vi "ELVIS III v1.0 AO Block Write Resource Manager.vi"(5 "DMA Resource":u8, 7 "Action":enum16{"Set", "Get"}(ring), 8 "error in (no error)":errorcluster, 10 "AO Resource In":T1={"AO FIFO Clock Divisor"=1000, "Wait Until Done?"=TRUE, "Write Mode"=0, "AO (N Samples) Configuration "=[]} caption="DO (N Samples) Configuration") -> (0 "error out":errorcluster, 1 "Action Succeeds":bool, 2 "AO Resource Out":T1={"AO FIFO Clock Divisor"=1000, "Wait Until Done?"=TRUE, "Write Mode"=0, "AO (N Samples) Configuration "=[]} caption="DO (N Samples) Configuration")   [LabVIEW 2021]
uses:
  <vilib>/myRIO/Common/Instrument Driver Framework/ELVIS III v1.0/AO Block/typedefs/ELVIS III AO Block Configuration.ctl
  <vilib>/myRIO/Common/Instrument Driver Framework/ELVIS III v1.0/AO Block/typedefs/ELVIS III AO Block Bank Data.ctl
  <vilib>/myRIO/Common/Instrument Driver Framework/myRIO v1.0/Resource Manager/vis/myRIO v1.0 Block Write Configuration.vi
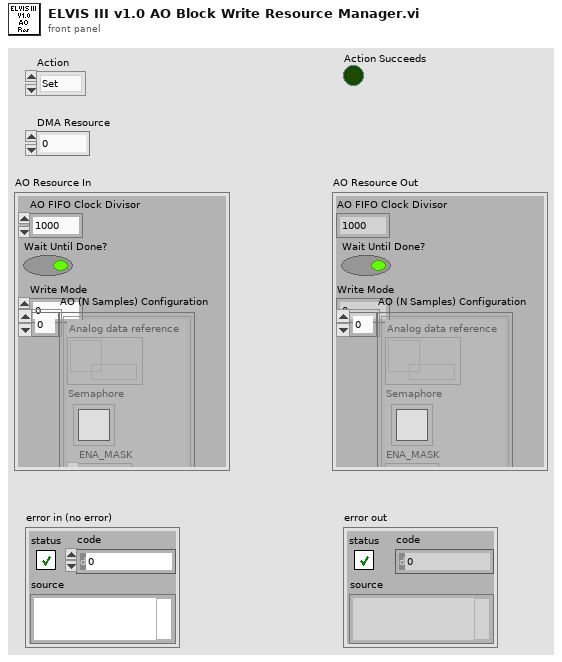
[diagram p1: front panel]
types:
  T1 = typedef "ELVIS III AO Block Configuration.ctl" = cluster{"AO FIFO Clock Divisor":u32, "Wait Until Done?":bool, "Write Mode":u8, "AO (N Samples) Configuration ":T2[]}
  T2 = typedef "ELVIS III AO Block Bank Data.ctl" = cluster{"Analog data reference":refnum<data-value>, "Semaphore":T3, "ENA_MASK":u8}
  T3 = typedef "Semaphore RefNum" = refnum<k1>
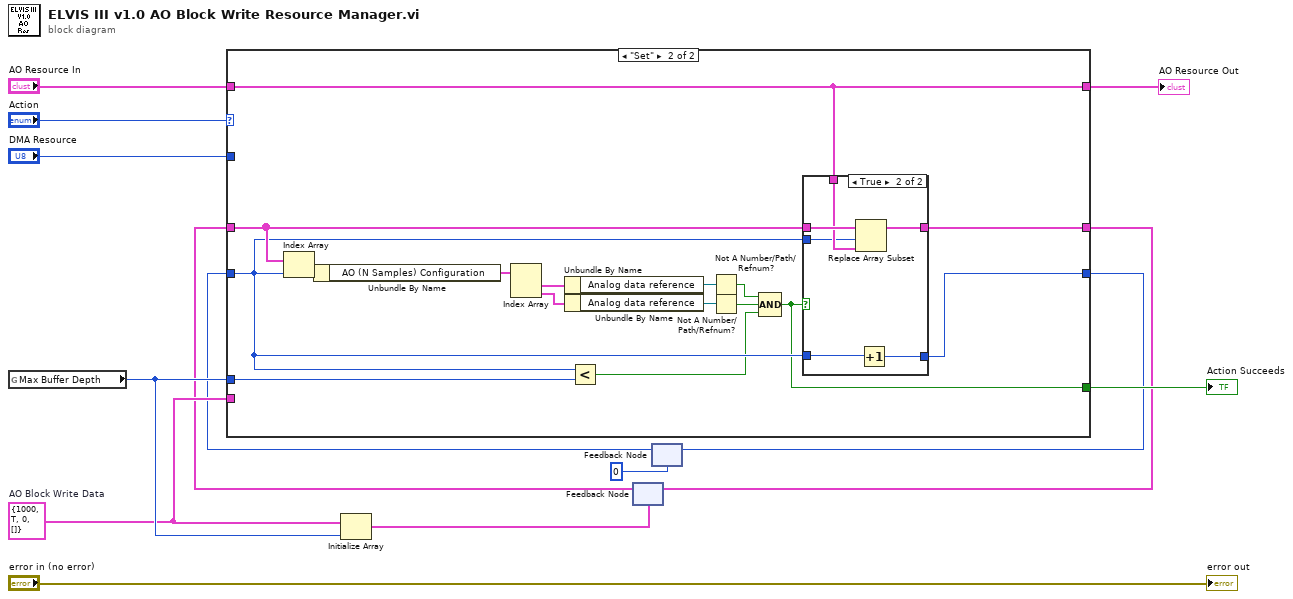
[diagram p0: block diagram]
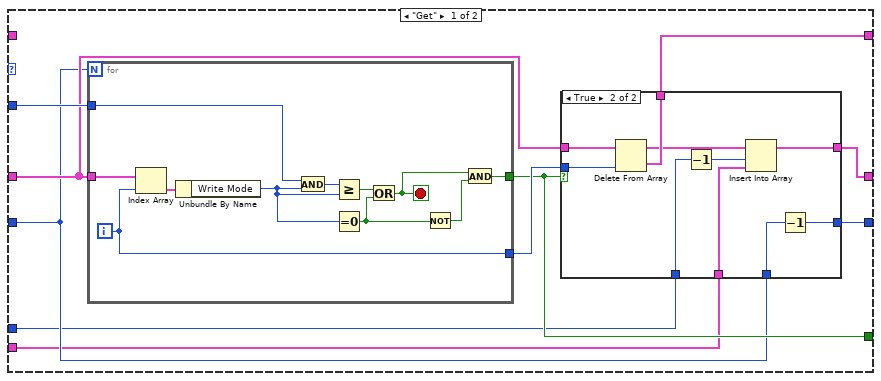
[diagram p2: hidden frame]
diagram:
  w10 = T1 {"AO FIFO Clock Divisor"=1000, "Wait Until Done?"=TRUE, "Write Mode"=0, "AO (N Samples) Configuration "=[]}  # AO Block Write Data
  n1 = global read "myRIO v1.0 Block Write Configuration.vi" "Max Buffer Depth"() -> (w13:u32)
  n2 = Initialize Array(w10, w13) -> (w6:T1[])
  n3 = feedback #1(w6) -> (w7:T1[])
  n4 = feedback #2(0) -> (w3:i32)
  n5 = case shown="\"Set\"" "Action" {
    tunnel: [w21 w57] -> w5
    tunnel: w7 -> [w22 w56]
    tunnel: "AO Resource In" -> [_ w52]
    tunnel: [w17 w55] -> w4
    tunnel: w13 -> [w16 w50]
    tunnel: w3 -> [w18 w51]
    tunnel: [w20 w48] -> w11
    tunnel: [w19 w52] -> w1
    tunnel: w10 -> [w15 _]
    tunnel: "DMA Resource" -> [w24 _]
    frame "Get" {
      n6 = for {
        N: w18 -> [_]
        tunnel: w22 -> [w46]
        tunnel: w24 -> [w45]
        tunnel: [w43] -> w23
        tunnel: [w38] -> w20
        i -> [w43]
        stop <- w40 stop-if-true
        n7 = Index Array(array=w46, index=w43) -> (element=w47:T1)
        n8 = Unbundle By Name(w47) -> ("Write Mode"=w42:u8)
        n9 = And(x=w45, y=w42) -> (x .and. y?=w37:u8)
        n10 = Greater Or Equal?(x=w37, y=w42) -> (x >= y?=w44:bool)
        n11 = Equal To 0?(x=w42) -> (x = 0?=w41:bool)
        n12 = Or(x=w44, y=w41) -> (x .or. y?=w40:bool)
        n13 = Not(x=w41) -> (.not. x?=w39:bool)
        n14 = And(x=w40, y=w39) -> (x .and. y?=w38:bool)
      }
      n15 = case shown="True" w20 {
        tunnel: w23 -> [_ w35]
        tunnel: w22 -> [w26 w36]
        tunnel: [w26 w27] -> w21
        tunnel: [_ w34] -> w19
        tunnel: w18 -> [w25 w33]
        tunnel: [w25 w32] -> w17
        tunnel: w16 -> [_ w30]
        tunnel: w15 -> [_ w28]
        frame False {
        }
        frame True {
          n16 = Delete From Array(array=w36, index=w35) -> (deleted portion=w34:T1, array with subset deleted=w31:T1[])  [unwired: 1 in]
          n17 = Decrement(x=w30) -> (x-1=w29:u32)
          n18 = Insert Into Array(array=w31, index=w29, new element=w28) -> (w27:T1[])
          n19 = Decrement(x=w33) -> (x-1=w32:i32)
        }
      }
    }
    frame "Set" {
      n20 = Index Array(array=w56, index=w51) -> (element=w60:T1)
      n21 = Unbundle By Name(w60) -> ("AO (N Samples) Configuration"=w63:T2[])
      n22 = Index Array(array=w63) -> (element #1=w62:T2, element #2=w61:T2)  [unwired: 2 in]
      n23 = Unbundle By Name(w62) -> ("Analog data reference"=w59:refnum<data-value>)
      n24 = Unbundle By Name(w61) -> ("Analog data reference"=w58:refnum<data-value>)
      n25 = Less?(x=w51, y=w50) -> (x < y?=w49:bool)
      n26 = Not A Number/Path/Refnum?(number/path/refnum=w59) -> (NaN/Path/Refnum?=w54:bool)
      n27 = Not A Number/Path/Refnum?(number/path/refnum=w58) -> (NaN/Path/Refnum?=w53:bool)
      n28 = Compound Arithmetic op=AND(w54, w53, w49) -> (w48:bool)
      n29 = case shown="True" w48 {
        tunnel: w56 -> [w65 w71]
        tunnel: [w65 w70] -> w57
        tunnel: w52 -> [_ w69]
        tunnel: [w64 w68] -> w55
        tunnel: w51 -> [w64 w67]
        tunnel: w51 -> [_ w66]
        frame False {
        }
        frame True {
          n30 = Replace Array Subset(array=w71, new element=w69, index=w66) -> (w70:T1[])
          n31 = Increment(x=w67) -> (x+1=w68:i32)
        }
      }
    }
  }
  "Action Succeeds" <- w11
  "AO Resource Out" <- w1
  n32 = feedback-in #1(w5) -> ()
  n33 = feedback-in #2(w4) -> ()
  "error out" <- "error in (no error)"
